vi "WriteGpsData.vi"(8 "Close File":bool, 9 "Path":path, 10 "Pathing Choice":bool, 11 "GPS Data":T1 {"Time"."GPS Time of Week" format="%.3f"; "Velocity, Correction & SET"."Extended Navigation Mode" items=["Non Differential"=0, "Code (RTCM Type 1 & 9)"=1, "Code, Single Frequency (WAAS)"=2, "Code, Dual Frequency (WAAS)"=3, "Code, Single Frequency (WCT)"=4, "Code/RCP, Dual Frequency (WCT)"=5, "Code, Single Frequency (RTG)"=6, "Code (RTCM Type 1 & 9) Dual Frequency"=10, "Code/RCP, Dual Frequency (RTG)"=11, "Code, Single Frequency (NCT-RTK)"=12, "Code, Single Frequency (RTCM 18 & 19)"=13, "Code, Single Frequency (RTCM 21 & 22)"=14, "Code, Single Frequency (CMR)"=15, "Code, Dual Frequency (NCT-RTK)"=16, "Code, Dual Frequency (RTCM 18 & 19)"=17, "Code, Dual Frequency (RTCM 20 & 21)"=18, "Code, Dual Frequency (CMR)"=19, "RTK (NCT-RTK)"=20, "RTK (RTCM 18 & 19)"=21, "RTK (RTCM 20 & 21)"=22, "RTK (CMR)"=23, "Code, Single Frequency with SET (RTG)"=24, "Code/RCP, Dual Frequency with SET (RTG)"=25, "RTK Extend"=26]}) -> ()   [LabVIEW 2011]
uses:
  WriteGpsDataGolbals.vi
  <vilib>/Utility/file.llb/Write To Spreadsheet File (DBL).vi
  <vilib>/Utility/file.llb/Write To Spreadsheet File (string).vi
panel:
  # "Auto Path"
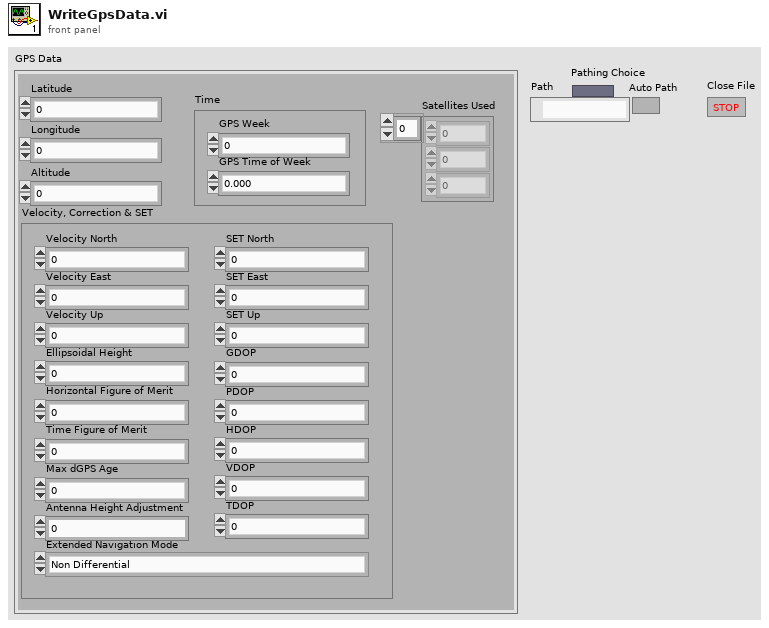
[diagram p1: front panel]
types:
  T1 = cluster{"Latitude":dbl, "Longitude":dbl, "Altitude":dbl, "Velocity, Correction & SET":cluster{"Velocity North":dbl, "Velocity East":dbl, "Velocity Up":dbl, "Ellipsoidal Height":dbl, "GDOP":sgl, "PDOP":sgl, "HDOP":sgl, "VDOP":sgl, "TDOP":sgl, "Horizontal Figure of Merit":u8, "Time Figure of Merit":u8, "Max dGPS Age":sgl, "Extended Navigation Mode":u8, "Antenna Height Adjustment ":dbl, "SET North":i32, "SET East":i32, "SET Up":i32}, "Time":cluster{"GPS Week":u16, "GPS Time of Week":sgl}, "Satellites Used":i32[]}
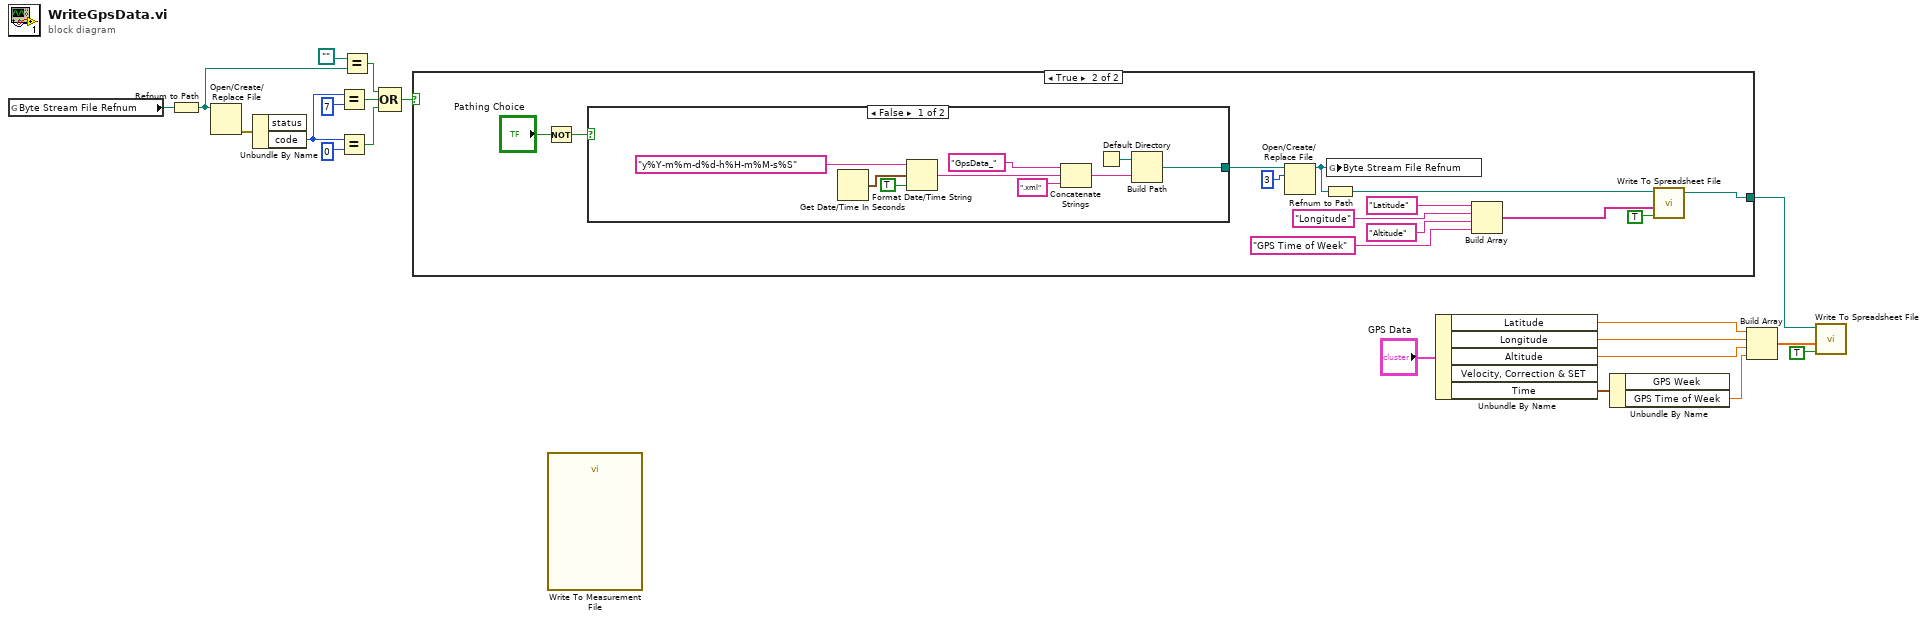
[diagram p0: block diagram]
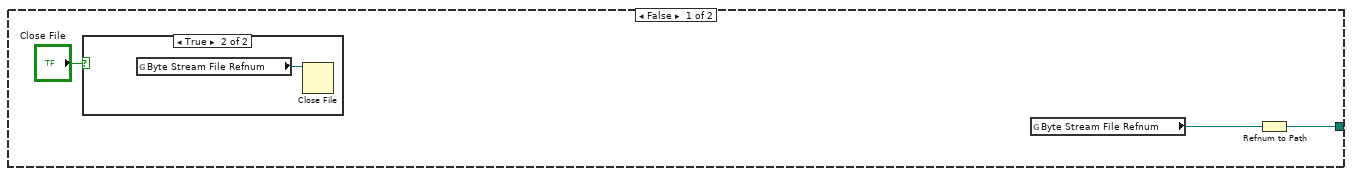
[diagram p2: hidden frame]
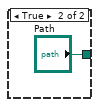
[diagram p4: hidden frame]
diagram:
  n1 = global read "WriteGpsDataGolbals.vi" "Byte Stream File Refnum"() -> (w12:refnum<file>)
  n2 = Refnum to Path(1:w12) -> (0:w3:path)
  n3 = Open/Create/Replace File(file path (use dialog)=w3) -> (error out=w6:errorcluster)  [unwired: 5 in, 2 out]
  n4 = Unbundle By Name(w6) -> ("code"=w5:i32)  [unwired: 1 out]
  n5 = Equal?(x=w5, y=7) -> (x = y?=w10:bool)
  n6 = Equal?(x=w5, y=0) -> (x = y?=w9:bool)
  n7 = Equal?(x=path "", y=w3) -> (x = y?=w2:bool)
  n8 = Compound Arithmetic op=OR(w2, w10, w9) -> (w11:bool)
  n9 = case shown="True" w11 {
    tunnel: [w22 w31] -> w1
    frame False {
      n10 = case shown="True" "Close File" {
        frame False {
        }
        frame True {
          n11 = global read "WriteGpsDataGolbals.vi" "Byte Stream File Refnum"() -> (w24:refnum<file>)
          n12 = Close File(refnum=w24) -> ()  [unwired: 1 in, 2 out]
        }
      }
      n13 = global read "WriteGpsDataGolbals.vi" "Byte Stream File Refnum"() -> (w21:refnum<file>)
      n14 = Refnum to Path(1:w21) -> (0:w22:path)
    }
    frame True {
      n15 = Not(x="Pathing Choice") -> (.not. x?=w35:bool)
      n16 = case shown="False" w35 {
        tunnel: [w38 "Path"] -> w34
        frame False {
          n17 = Get Date/Time In Seconds() -> (seconds since 1Jan1904=w45:timestamp)
          n18 = Format Date/Time String(time format string (%c)="y%Y-m%m-d%d-h%H-m%M-s%S", seconds (now)=w45, UTC format=TRUE) -> (date/time string=w43:string)
          n19 = Concatenate Strings("GpsData_", w43, ".xml") -> (w39:string)
          n20 = Default Directory() -> (w40:path)
          n21 = Build Path(base path=w40, name or relative path=w39) -> (appended path=w38:path)
        }
        frame True {
        }
      }
      n22 = Open/Create/Replace File(file path (use dialog)=w34, operation (0:open)=3) -> (refnum out=w25:refnum<file>)  [unwired: 4 in, 2 out]
      n23 = Refnum to Path(1:w25) -> (0:w32:path)
      n24 = global write "WriteGpsDataGolbals.vi" "Byte Stream File Refnum"(w25) -> ()
      n25 = Build Array("Latitude", "Longitude", "Altitude", "GPS Time of Week") -> (w26:string[])
      n26 = call-poly <vilib>:"Write To Spreadsheet File.vi"("append to file? (new file:F)"=TRUE, "1D data"=w26, "file path (dialog if empty)"=w32) -> ("new file path (Not A Path if cancelled)"=w31:path)  [unwired: 5 in]
    }
  }
  n27 = call "Write To Measurement File"() -> ()  [unwired: 17 in, 3 out]
  n28 = Unbundle By Name("GPS Data") -> ("Latitude"=w15:dbl, "Longitude"=w17:dbl, "Altitude"=w16:dbl, "Time"=w19:cluster{"GPS Week":u16, "GPS Time of Week":sgl})  [unwired: 1 out]
  n29 = Unbundle By Name(w19) -> ("GPS Time of Week"=w20:sgl)  [unwired: 1 out]
  n30 = Build Array(w15, w17, w16, w20) -> (w18:dbl[])
  n31 = call-poly <vilib>:"Write To Spreadsheet File.vi"("append to file? (new file:F)"=TRUE, "1D data"=w18, "file path (dialog if empty)"=w1) -> ()  [unwired: 5 in, 1 out]
